vi "Set State.vi"(7 "VI Ref":refnum<vi>, 8 "Error":errorcluster, 9 "State":T1(ring)=enum."Standard", 11 "FP":refnum<class "FP.lvclass">) -> (0 "Error Out":errorcluster, 3 "FP Out":refnum<class "FP.lvclass">, 5 "VI Ref":refnum<vi>)   [LabVIEW 2025, in "FP.lvclass"]
uses:
  FP.lvclass
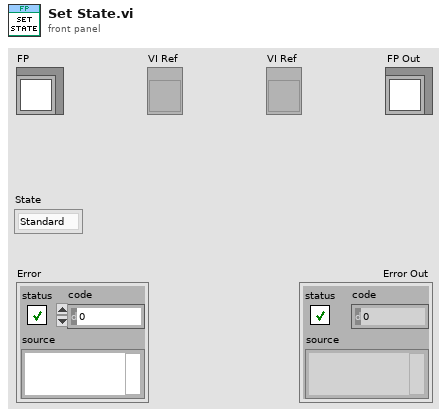
[diagram p1: front panel]
types:
  T1 = enum32{"Invalid", "Standard", "Closed", "Hidden", "Minimized", "Maximized"}
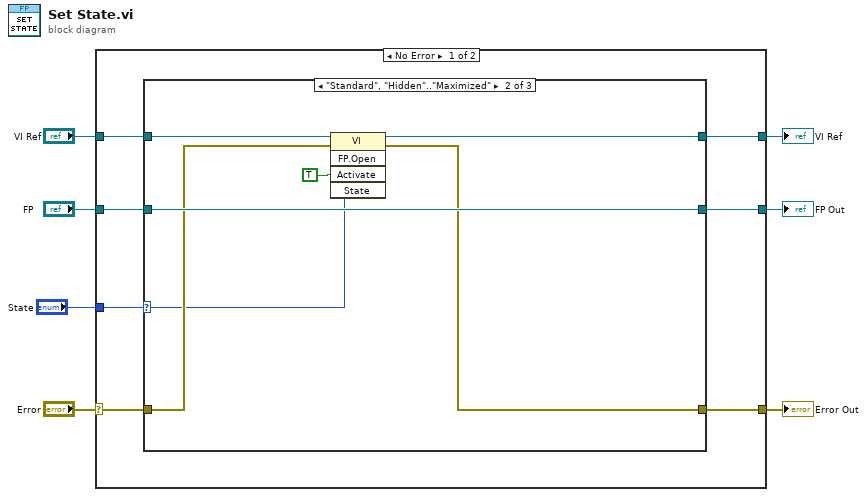
[diagram p0: block diagram]
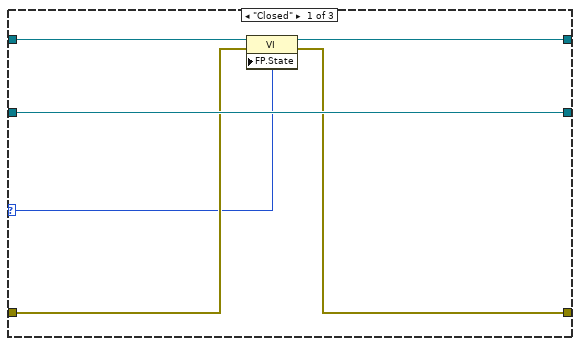
[diagram p2: hidden frame]
diagram:
  n1 = case shown="No Error" "Error" {
    selector: "Error" -> [w14 w33]
    tunnel: [w9 w33] -> w6
    tunnel: [w10 w32] -> w4
    tunnel: "FP" -> [w13 w32]
    tunnel: "VI Ref" -> [w12 w31]
    tunnel: [w11 w31] -> w2
    tunnel: "State" -> [w8 _]
    frame No Error {
      n2 = case shown="\"Standard\", \"Hidden\"..\"Maximized\"" w8 {
        selector: w8 -> [w15 w23 _]
        tunnel: w14 -> [w17 w26 w28]
        tunnel: w13 -> [w20 w27 w30]
        tunnel: w12 -> [w19 w21 w29]
        tunnel: [w18 w24 w29] -> w11
        tunnel: [w20 w27 w30] -> w10
        tunnel: [w16 w25 w28] -> w9
        frame "Closed" {
          n3 = property class="VI"(reference=w19, error in=w17, "FP.State"=w15) -> (reference out=w18:refnum<vi>, error out=w16:errorcluster)
        }
        frame "Standard", "Hidden".."Maximized" {
          n4 = invoke class="VI" method="FP.Open"(reference=w21, error in=w26, "Activate"=TRUE ("Activate?"), "State"=w23) -> (reference out=w24:refnum<vi>, error out=w25:errorcluster)  [unwired: 1 in, 3 out]
        }
        frame "Invalid" {
        }
      }
    }
    frame Error {
    }
  }
  "Error Out" <- w6
  "FP Out" <- w4
  "VI Ref" <- w2
